vi "Write Power FIFO.vi"(4 "T_Out":u64, 6 "T0":u64, 8 "error in (no error)":errorcluster, 9 "Timeout (ms)":i32=100, 10 "Data In":T1[](array[typedef])=[{"measurement"=[], "dT"=0.0, "Timestamp"=0}, {"measurement"=[], "dT"=0.0, "Timestamp"=0}], 11 "CIFTag in":refnum<class "CIF_NIChn_Fifo_Power.lvclass">) -> (0 "error out":errorcluster, 1 "timed out?":bool, 2 "Data Out":T1[](array[typedef]), 3 "CIFTag out":refnum<class "CIF_NIChn_Fifo_Power.lvclass">)   [LabVIEW 2021, in "CIF_NIChn_Fifo_Power.lvclass"]
uses:
  CIF_NIChn_Fifo_Power.lvclass
  D:/dev/CIF-LVCore/src/Channels/CIFChannels/CIFChannels.lvclass
  D:/dev/CIF-LVCore/src/Channels/CIF_NIChn/NIChn/CIF_NIChn.lvclass
  ChannelCommon/typedef/Datatype Waveform.ctl
  CIFChannels/CIFChannels.lvclass/CIFChannels.ctl
  CIF_NIChn_Fifo_Power.lvclass/CIF_NIChn_Fifo_Power.ctl
  ChannelCommon/CIFFIFO/CIFfifo.lvclass/CIFfifo.ctl
  NIChn/CIF_NIChn.lvclass/CIF_NIChn.ctl
  ChannelCommon/CIFFIFO/Accessors/Read Length.vi
  CIFCore/Common/Utilities/Append Error Location.vi
  <vilib>/CIFChannels/SubVIs/Get dll Path.vi
  ChannelCommon/CIFFIFO/Utilities/Update Header.vi
  ChannelCommon/Utilities/Flatten Header.vi
  ChannelCommon/Flatten/trash_Waveform Flatten.vi
  ChannelCommon/CIFFIFO/Accessors/Write T0.vi
  ChannelCommon/CIFFIFO/Accessors/Write T_Out.vi
  ChannelCommon/CIFFIFO/Accessors/Write Payload Length.vi
  ChannelCommon/CIFFIFO/Accessors/Read Header.vi
  ChannelCommon/CIFFIFO/Accessors/Write Header.vi
  CIFChannels/Accessors/Read ClockID.vi
  ChannelCommon/Flatten/trash_Waveform Flatten.vi/e2488641-f297-4923-bbd0-3c2628a14485.vi
  ChannelCommon/Flatten/trash_Waveform Flatten.vi/b4043d5f-ec85-461b-bf30-5d9c9f378a85.vi
  ChannelCommon/Flatten/trash_Waveform Flatten.vi/7a03eb27-3fd6-4af7-b359-0d2263a4e3bc.vi
  ChannelCommon/Flatten/trash_Waveform Flatten.vi/e2488641-f297-4923-bbd0-3c2628a14485.vi/c28b0ead-42ad-4072-80a2-aca7f2bd7ce3.vi
  ChannelCommon/Flatten/trash_Waveform Flatten.vi/b4043d5f-ec85-461b-bf30-5d9c9f378a85.vi/c28b0ead-42ad-4072-80a2-aca7f2bd7ce3.vi
  ChannelCommon/Flatten/trash_Waveform Flatten.vi/7a03eb27-3fd6-4af7-b359-0d2263a4e3bc.vi/c28b0ead-42ad-4072-80a2-aca7f2bd7ce3.vi
  ChannelCommon/Utilities/Update Time.vi
  NIChn/CIF_NIChn.lvclass
  <vilib>/CIFChannels/CIFChannelCore.lvlib
  ChannelCommon/CIFFIFO/CIFfifo.lvclass
  ChannelCommon/ChannelCommon.lvlib
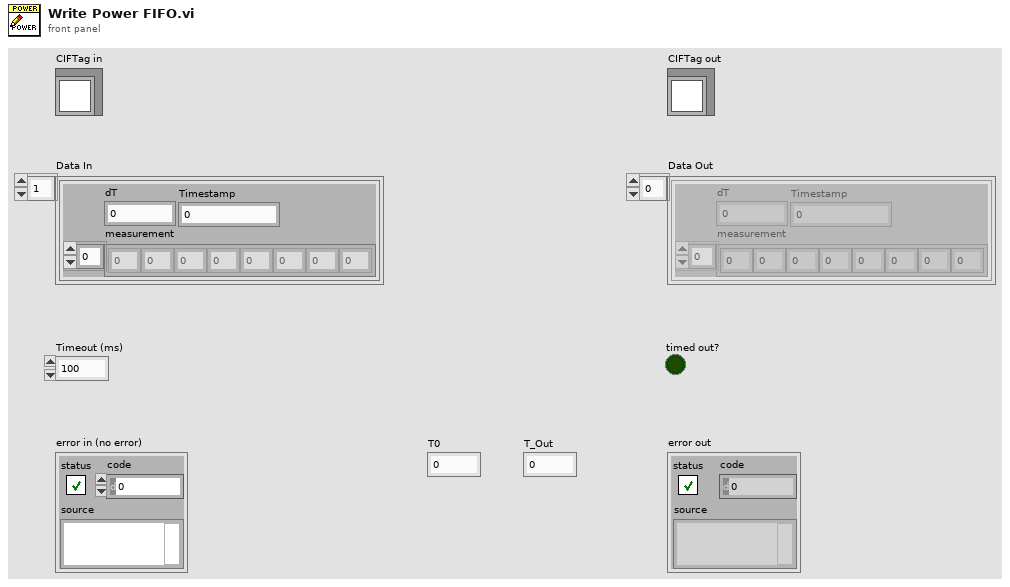
[diagram p1: front panel]
types:
  T1 = typedef "ChannelCommon.lvlib/Datatype Waveform.ctl" = cluster{"measurement":dbl[], "dT":dbl, "Timestamp":u64}
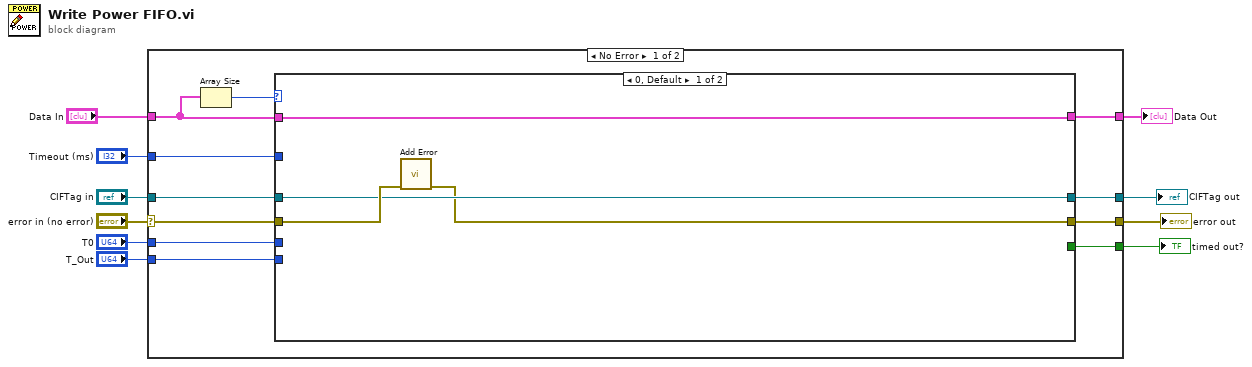
[diagram p0: block diagram]
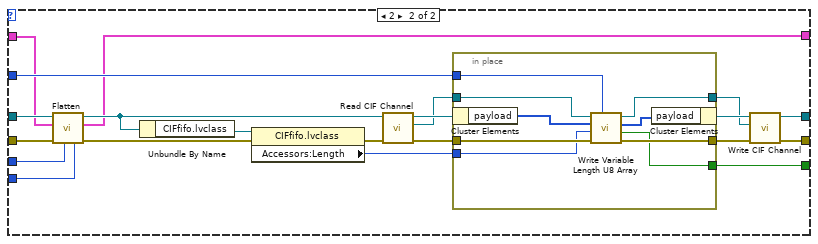
[diagram p2: hidden frame]
diagram:
  n1 = case shown="No Error" "error in (no error)" {
    selector: "error in (no error)" -> [w16 w58]
    tunnel: [w18 w58] -> w9
    tunnel: [w20 w57] -> w7
    tunnel: "CIFTag in" -> [w17 w57]
    tunnel: [w21 _] -> w6
    tunnel: "Timeout (ms)" -> [w19 _]
    tunnel: "T_Out" -> [w14 _]
    tunnel: "T0" -> [w15 _]
    tunnel: [w13 w56] -> w2
    tunnel: "Data In" -> [w12 w56]
    frame No Error {
      n2 = Array Size(array=w12) -> (size(s)=w11:i32)
      n3 = case shown="0, Default" w11 {
        tunnel: [_ w46] -> w21
        tunnel: [w24 w42] -> w20
        tunnel: w19 -> [_ w38]
        tunnel: [w23 w37] -> w18
        tunnel: w17 -> [w24 w34]
        tunnel: w16 -> [w25 w31]
        tunnel: w15 -> [_ w30]
        tunnel: w14 -> [_ w29]
        tunnel: [w22 w27] -> w13
        tunnel: w12 -> [w22 w26]
        frame 0, Default {
          n4 = call "Add Error.vi"("error in (no error)"=w25) -> ("error out"=w23:errorcluster)  [unwired: 10 in]
        }
        frame 2 {
          n5 = call "Flatten.vi"("T_Out"=w29, "T0"=w30, "error in (no error)"=w31, "Data"=w26, "CIFTag in"=w34) -> ("error out"=w32:errorcluster, "Data out"=w27:T1[], "CIFTag out"=w33:refnum<class "CIF_NIChn_Fifo_Power.lvclass">)  [unwired: 4 in]
          n6 = Unbundle By Name(w33) -> ("CIFfifo.lvclass"=w36:refnum<class "CIFfifo.lvclass">)
          n7 = property class="CIFfifo.lvclass"(reference=w36, error in=w32) -> (error out=w35:errorcluster, "Accessors:Length"=w28:u64)  [unwired: 1 out]
          n8 = call "Read CIF Channel.vi"("error in (no error)"=w35, "CIFTag in"=w33) -> ("error out"=w44:errorcluster, "CIF Channel"=w40:refnum<k21>, "CIFTag out"=w45:refnum<class "CIF_NIChn_Fifo_Power.lvclass">)  [unwired: 7 in]
          n9 = in-place {
            in-place-border: w44 -> [w55]
            in-place-border: [w54] -> w41
            in-place-border: [w53] -> w46
            in-place-border: w40 -> [w52]
            in-place-border: [w51] -> w39
            in-place-border: w38 -> [w50]
            in-place-border: w28 -> [w48]
            n10 = in-place-cluster #1(w45) -> ("payload"=w49:u8[])
            n11 = call <vilib>:"Write Variable Length U8 Array.vi"("Timeout (ms)"=w50, "error in"=w55, "numElements"=w48, "U8 Array in"=w49, "CIF Channel in"=w52) -> ("error out"=w54:errorcluster, "Timed out?"=w53:bool, "U8 Array out"=w47:u8[], "CIF Channel out"=w51:refnum<k21>)  [unwired: 3 in]
            n12 = in-place-cluster #1("payload"=w47) -> (w43:refnum<class "CIF_NIChn_Fifo_Power.lvclass">)
          }
          n13 = call "Write CIF Channel.vi"("error in (no error)"=w41, "CIF Channel"=w39, "CIFTag in"=w43) -> ("error out"=w37:errorcluster, "CIFTag out"=w42:refnum<class "CIF_NIChn_Fifo_Power.lvclass">)  [unwired: 7 in]
        }
      }
    }
    frame Error {
    }
  }
  "error out" <- w9
  "CIFTag out" <- w7
  "timed out?" <- w6
  "Data Out" <- w2
